vi "VCO-FM.vi"() -> ()   [LabVIEW 2012]
uses:
  <vilib>/rvi/FXPMathLib/basic elements/FxpIntAccumulator/subVIs/nifxpmath_IntAccumulator_SimConfig.ctl
  <vilib>/rvi/FXPMathLib/FxpSinAndCos/subVIs/nifxpmath_SinAndCos_SimConfig.ctl
  <vilib>/rvi/eio/common/nirviEmuTemplateMethod_errors.vi
  <vilib>/rvi/interface/RandomDataEmulation/nirviRandomDataFPGAFIFO.vi
  <vilib>/rvi/interface/RandomDataEmulation/niFpgaRandomDataHandleErrors.vi
  <vilib>/rvi/FXPMathLib/basic elements/FxpIntAccumulator/simVIs/DllFxpIntAccumulator_sub.vi
  <vilib>/rvi/FXPMathLib/FxpSinAndCos/simVIs/DllFxpSinAndCosTemp_sub.vi
  <vilib>/eio/EIONode/EIONode.xnode
  <vilib>/rvi/DataTransferAndStorage/Container/XNode/niFpgaContainer.xnode
  <vilib>/rvi/interface/RandomDataEmulation/nirviRandomDataFpgaReadWriteTemplate.vi
  <vilib>/rvi/FXPMathLib/basic elements/FxpIntAccumulator/XNode/nifxpmath_IntAccumulator.xnode
  <vilib>/rvi/FXPMathLib/FxpSinAndCos/XNode/nifxpmath_SinAndCos.xnode
panel:
  in  "Angular Frequency":fxp<+/-,22,22>
  out "Ticks":i16
  in  "DAQ Acquisition Rate":i16
  out "Test Input":fxp<+/-,64,32>
  out "Sine Output":fxp<+/-,64,32>
  in  "Voltage (V)":fxp<+,64,12>=3276.8125
  out "Numeric":fxp<+/-,64,32>
  out "Summation":fxp<+/-,64,32>
  out "Z":fxp<+/-,64,32>
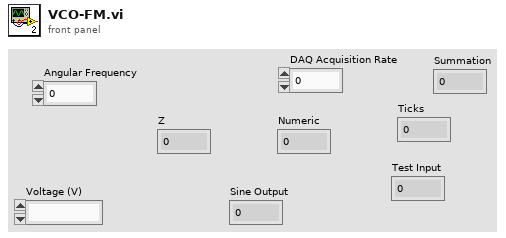
[diagram p1: front panel]
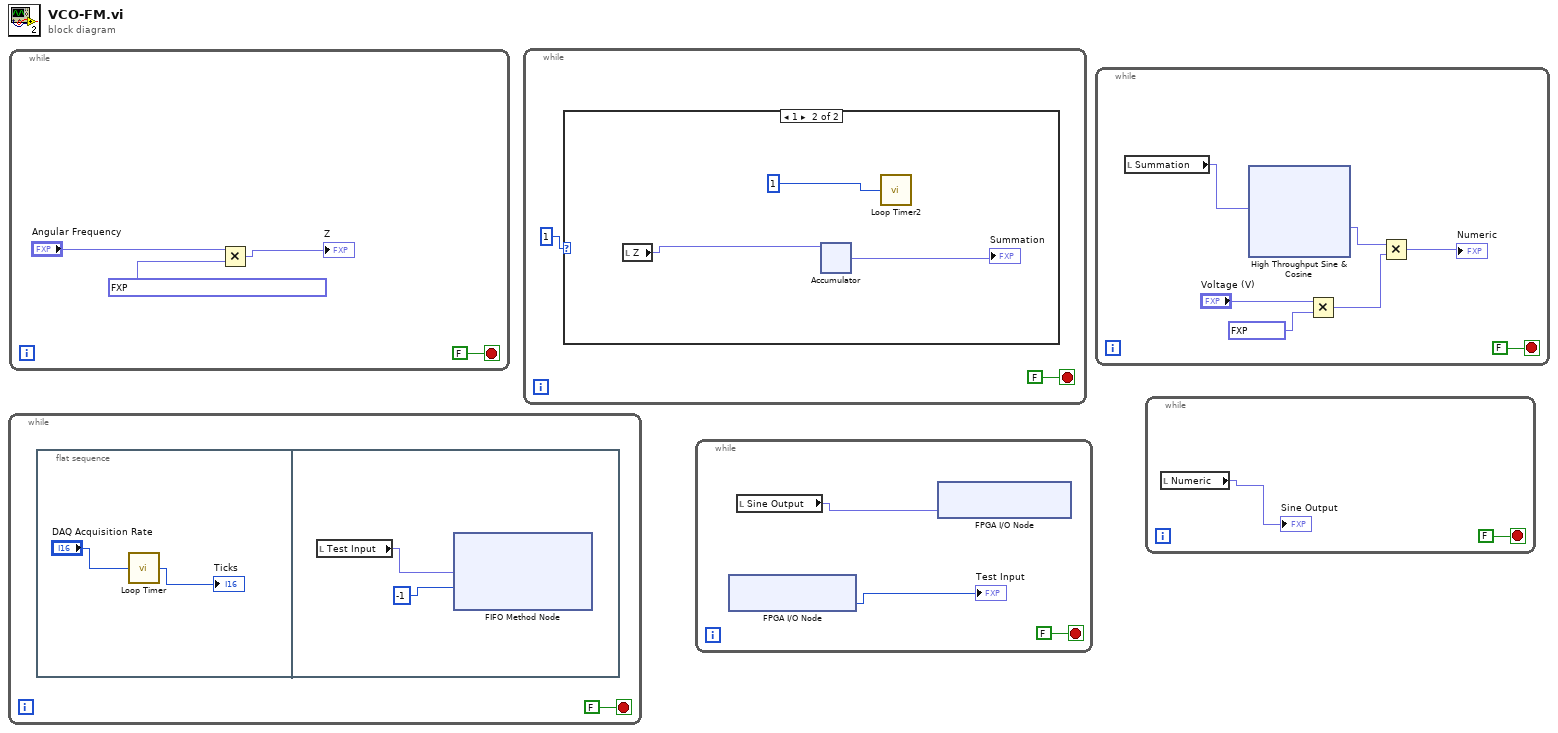
[diagram p0: block diagram]
diagram:
  n1 = while {
    stop <- FALSE stop-if-true
    n2 = flat-sequence {
      frame #0 {
        n3 = call "Loop Timer"("Count(uSec)"="DAQ Acquisition Rate") -> ("Tick Count(uSec)"=→"Ticks":u32)
      }
      frame #1 {
        n4 = local read "Test Input"() -> (w5:fxp<+/-,64,32>)
        n5 = xnode ("FIFO Method Node")("Element"=w5, "Timeout"=-1) -> ()  [unwired: 1 in, 2 out]
      }
    }
  }
  n6 = while {
    stop <- FALSE stop-if-true
    n7 = Multiply(x="Angular Frequency", y=fxp<+,46,7> 1.0000003385357559e-06) -> (x*y=→"Z":fxp<+/-,64,29>)
  }
  n8 = while {
    stop <- FALSE stop-if-true
    n9 = case shown="1" 1 {
      frame 0, Default {
      }
      frame 1 {
        n10 = local read "Z"() -> (w14:fxp<+/-,64,32>)
        n11 = xnode "Accumulator"("x"=w14) -> ("s"=→"Summation":fxp<+/-,64,32>)  [unwired: 4 in, 1 out]
        n12 = call "Loop Timer2"("Count(uSec)"=1) -> ()  [unwired: 1 out]
      }
    }
  }
  n13 = while {
    stop <- FALSE stop-if-true
    n14 = xnode "FPGA I/O Node"() -> ("Connector0/AI6"=→"Test Input":i16)  [unwired: 1 in, 1 out]
    n15 = local read "Sine Output"() -> (w43:fxp<+/-,64,32>)
    n16 = xnode "FPGA I/O Node"("Connector0/AO2"=w43) -> ()  [unwired: 1 in, 1 out]
  }
  n17 = while {
    stop <- FALSE stop-if-true
    n18 = local read "Summation"() -> (w50:fxp<+/-,64,32>)
    n19 = xnode "High Throughput Sine & Cosine"("x (pi)"=w50) -> ("sin(x)"=w49:fxp<+/-,16,2>)  [unwired: 1 out]
    n20 = Multiply(x="Voltage (V)", y=fxp<+,17,12> 3276.8125) -> (x*y=w45:fxp<+,64,24>)
    n21 = Multiply(x=w49, y=w45) -> (x*y=→"Numeric":fxp<+/-,64,26>)
  }
  n22 = while {
    stop <- FALSE stop-if-true
    n23 = local read "Numeric"() -> (→"Sine Output":fxp<+/-,64,32>)
  }
